vi "canDataSort.vi"() -> ()   [LabVIEW 2023] (continued)
\tFF\r\n      1212  1FFFFFFF   00000004    8        00\t20\tFF\tFF\tFF\tFF\tFF\tFF\r\n      1203  0CF102A7   00000004    8        30\t75\tE0\t2E\t80\tFF\tFF\tFD\r\n      1203  0CF101A7   00000004    8        68\t00\t97\tCC\t00\t15\t39\t56\r\n      1202  1FFFFFFF   00000004    8        00\t00\tFF\tFF\tFF\tFF\tFF\tFF\r\n      1243  0C3C4D4A   00000004    8        BE\tFF\tFF\t7F\t18\tFF\tFF\t44\r\n      1243  0CF101A7   00000004    8        68\t00\t97\tCC\t00\t16\t39\t58\r\n      1242  18F120F0   00000004    8        2B\t75\t60\tB1\tB0\t01\tFF\tFF\r\n      1241  18F11FF0   00000004    8        FF\t3F\t90\t68\t88\t1B\t10\t4C\r\n      1232  1FFFFFFF   00000004    8        00\t20\tFF\tFF\tFF\tFF\tFF\tFF\r\n      1223  0CF102A7   00000004    8        30\t75\tE0\t2E\t80\tFF\tFF\tFD\r\n      1223  0CF101A7   00000004    8        68\t00\t97\tCC\t00\t16\t39\t57\r\n      1222  1FFFFFFF   00000004    8        00\t00\tFF\tFF\tFF\tFF\tFF\tFF\r\n      1212  1FFFFFFF   00000004    8        00\t20\tFF\tFF\tFF\tFF\tFF\tFF\r\n      1203  0CF102A7   00000004    8        30\t75\tE0\t2E\t80\tFF\tFF\tFD\r\n      1203  0CF101A7   00000004    8        68\t00\t97\tCC\t00\t15\t39\t56\r\n      1244  0CF102A7   00000004    8        30\t75\tE0\t2E\t80\tFF\tFF\tFD\r\n      1243  0C3C4D4A   00000004    8        BE\tFF\tFF\t7F\t18\tFF\tFF\t44\r\n      1243  0CF101A7   00000004    8        68\t00\t97\tCC\t00\t16\t39\t58\r\n      1242  18F120F0   00000004    8        2B\t75\t60\tB1\tB0\t01\tFF\tFF\r\n      1241  18F11FF0   00000004    8        FF\t3F\t90\t68\t88\t1B\t10\t4C\r\n      1232  1FFFFFFF   00000004    8        00\t20\tFF\tFF\tFF\tFF\tFF\tFF\r\n      1223  0CF102A7   00000004    8        30\t75\tE0\t2E\t80\tFF\tFF\tFD\r\n      1223  0CF101A7   00000004    8        68\t00\t97\tCC\t00\t16\t39\t57\r\n      1222  1FFFFFFF   00000004    8        00\t00\tFF\tFF\tFF\tFF\tFF\tFF\r\n      1212  1FFFFFFF   00000004    8        00\t20\tFF\tFF\tFF\tFF\tFF\tFF\r\n      1203  0CF102A7   00000004    8        30\t75\tE0\t2E\t80\tFF\tFF\tFD\r\n      1244  0CF103A7   00000004    8        17\t1F\t08\t60\tB1\t1F\t08\t44\r\n      1244  0CF102A7   00000004    8        30\t75\tE0\t2E\t80\tFF\tFF\tFD\r\n      1243  0C3C4D4A   00000004    8        BE\tFF\tFF\t7F\t18\tFF\tFF\t44\r\n      1243  0CF101A7   00000004    8        68\t00\t97\tCC\t00\t16\t39\t58\r\n      1242  18F120F0   00000004    8        2B\t75\t60\tB1\tB0\t01\tFF\tFF\r\n      1241  18F11FF0   00000004    8        FF\t3F\t90\t68\t88\t1B\t10\t4C\r\n      1232  1FFFFFFF   00000004    8        00\t20\tFF\tFF\tFF\tFF\tFF\tFF\r\n      1223  0CF102A7   00000004    8        30\t75\tE0\t2E\t80\tFF\tFF\tFD\r\n      1223  0CF101A7   00000004    8        68\t00\t97\tCC\t00\t16\t39\t57\r\n      1222  1FFFFFFF   00000004    8        00\t00\tFF\tFF\tFF\tFF\tFF\tFF\r\n      1212  1FFFFFFF   00000004    8        00\t20\tFF\tFF\tFF\tFF\tFF\tFF\r\n      1245  0CF104A7   00000004    8        F0\t60\t22\tFC\tFF\tFF\tFF\t44\r\n      1244  0CF103A7   00000004    8        17\t1F\t08\t60\tB1\t1F\t08\t44\r\n      1244  0CF102A7   00000004    8        30\t75\tE0\t2E\t80\tFF\tFF\tFD\r\n      1243  0C3C4D4A   00000004    8        BE\tFF\tFF\t7F\t18\tFF\tFF\t44\r\n      1243  0CF101A7   00000004    8        68\t00\t97\tCC\t00\t16\t39\t58\r\n      1242  18F120F0   00000004    8        2B\t75\t60\tB1\tB0\t01\tFF\tFF\r\n      1241  18F11FF0   00000004    8        FF\t3F\t90\t68\t88\t1B\t10\t4C\r\n      1232  1FFFFFFF   00000004    8        00\t20\tFF\tFF\tFF\tFF\tFF\tFF\r\n      1223  0CF102A7   00000004    8        30\t75\tE0\t2E\t80\tFF\tFF\tFD\r\n      1223  0CF101A7   00000004    8        68\t00\t97\tCC\t00\t16\t39\t57\r\n      1222  1FFFFFFF   00000004    8        00\t00\tFF\tFF\tFF\tFF\tFF\tFF\r\n      1245  18F106A7   00000004    8        00\tF7\tFF\tFF\tFF\tFF\tFF\t89\r\n      1245  0CF104A7   00000004    8        F0\t60\t22\tFC\tFF\tFF\tFF\t44\r\n      1244  0CF103A7   00000004    8        17\t1F\t08\t60\tB1\t1F\t08\t44\r\n      1244  0CF102A7   00000004    8        30\t75\tE0\t2E\t80\tFF\tFF\tFD\r\n      1243  0C3C4D4A   00000004    8        BE\tFF\tFF\t7F\t18\tFF\tFF\t44\r\n      1243  0CF101A7   00000004    8        68\t00\t97\tCC\t00\t16\t39\t58\r\n      1242  18F120F0   00000004    8        2B\t75\t60\tB1\tB0\t01\tFF\tFF\r\n      1241  18F11FF0   00000004    8        FF\t3F\t90\t68\t88\t1B\t10\t4C\r\n      1232  1FFFFFFF   00000004    8        00\t20\tFF\tFF\tFF\tFF\tFF\tFF\r\n      1223  0CF102A7   00000004    8        30\t75\tE0\t2E\t80\tFF\tFF\tFD\r\n      1223  0CF101A7   00000004    8        68\t00\t97\tCC\t00\t16\t39\t57\r\n      1246  18F121F0   00000004    8        09\t18\t00\t00\tFF\tFF\tB0\t01\r\n      1245  18F106A7   00000004    8        00\tF7\tFF\tFF\tFF\tFF\tFF\t89\r\n      1245  0CF104A7   00000004    8        F0\t60\t22\tFC\tFF\tFF\tFF\t44\r\n      1244  0CF103A7   00000004    8        17\t1F\t08\t60\tB1\t1F\t08\t44\r\n      1244  0CF102A7   00000004    8        30\t75\tE0\t2E\t80\tFF\tFF\tFD\r\n      1243  0C3C4D4A   00000004    8        BE\tFF\tFF\t7F\t18\tFF\tFF\t44\r\n      1243  0CF101A7   00000004    8        68\t00\t97\tCC\t00\t16\t39\t58\r\n      1242  18F120F0   00000004    8        2B\t75\t60\tB1\tB0\t01\tFF\tFF\r\n      1241  18F11FF0   00000004    8        FF\t3F\t90\t68\t88\t1B\t10\t4C\r\n      1232  1FFFFFFF   00000004    8        00\t20\tFF\tFF\tFF\tFF\tFF\tFF\r\n      1223  0CF102A7   00000004    8        30\t75\tE0\t2E\t80\tFF\tFF\tFD\r\n      1247  1FFFFFFF   00000004    8        00\t20\tFF\tFF\tFF\tFF\tFF\tFF\r\n      1246  18F121F0   00000004    8        09\t18\t00\t00\tFF\tFF\tB0\t01\r\n      1245  18F106A7   00000004    8        00\tF7\tFF\tFF\tFF\tFF\tFF\t89\r\n      1245  0CF104A7   00000004    8        F0\t60\t22\tFC\tFF\tFF\tFF\t44\r\n      1244  0CF103A7   00000004    8        17\t1F\t08\t60\tB1\t1F\t08\t44\r\n      1244  0CF102A7   00000004    8        30\t75\tE0\t2E\t80\tFF\tFF\tFD\r\n      1243  0C3C4D4A   00000004    8        BE\tFF\tFF\t7F\t18\tFF\tFF\t44\r\n      1243  0CF101A7   00000004    8        68\t00\t97\tCC\t00\t16\t39\t58\r\n      1242  18F120F0   00000004    8        2B\t75\t60\tB1\tB0\t01\tFF\tFF\r\n      1241  18F11FF0   00000004    8        FF\t3F\t90\t68\t88\t1B\t10\t4C\r\n      1232  1FFFFFFF   00000004    8        00\t20\tFF\tFF\tFF\tFF\tFF\tFF\r\n      1252  1FFFFFFF   00000004    8        00\t20\tFF\tFF\tFF\tFF\tFF\tFF\r\n      1247  1FFFFFFF   00000004    8        00\t20\tFF\tFF\tFF\tFF\tFF\tFF\r\n      1246  18F121F0   00000004    8        09\t18\t00\t00\tFF\tFF\tB0\t01\r\n      1245  18F106A7   00000004    8        00\tF7\tFF\tFF\tFF\tFF\tFF\t89\r\n      1245  0CF104A7   00000004    8        F0\t60\t22\tFC\tFF\tFF\tFF\t44\r\n      1244  0CF103A7   00000004    8        17\t1F\t08\t60\tB1\t1F\t08\t44\r\n      1244  0CF102A7   00000004    8        30\t75\tE0\t2E\t80\tFF\tFF\tFD\r\n      1243  0C3C4D4A   00000004    8        BE\tFF\tFF\t7F\t18\tFF\tFF\t44\r\n      1243  0CF101A7   00000004    8        68\t00\t97\tCC\t00\t16\t39\t58\r\n      1242  18F120F0   00000004    8        2B\t75\t60\tB1\tB0\t01\tFF\tFF\r\n      1241  18F11FF0   00000004    8        FF\t3F\t90\t68\t88\t1B\t10\t4C\r\n      1262  1FFFFFFF   00000004    8        00\t00\tFF\tFF\tFF\tFF\tFF\tFF\r\n      1252  1FFFFFFF   00000004    8        00\t20\tFF\tFF\tFF\tFF\tFF\tFF\r\n      1247  1FFFFFFF   00000004    8        00\t20\tFF\tFF\tFF\tFF\tFF\tFF\r\n      1246  18F121F0   00000004    8        09\t18\t00\t00\tFF\tFF\tB0\t01\r\n      1245  18F106A7   00000004    8        00\tF7\tFF\tFF\tFF\tFF\tFF\t89\r\n      1245  0CF104A7   00000004    8        F0\t60\t22\tFC\tFF\tFF\tFF\t44\r\n      1244  0CF103A7   00000004    8        17\t1F\t08\t60\tB1\t1F\t08\t44\r\n      1244  0CF102A7   00000004    8        30\t75\tE0\t2E\t80\tFF\tFF\tFD\r\n      1243  0C3C4D4A   00000004    8        BE\tFF\tFF\t7F\t18\tFF\tFF\t44\r\n      1243  0CF101A7   00000004    8        68\t00\t97\tCC\t00\t16\t39\t58\r\n      1242  18F120F0   00000004    8        2B\t75\t60\tB1\tB0\t01\tFF\tFF\r\n      1263  0CF101A7   00000004    8        68\t00\t97\tCC\t00\t16\t39\t59\r\n      1262  1FFFFFFF   00000004    8        00\t00\tFF\tFF\tFF\tFF\tFF\tFF\r\n      1252  1FFFFFFF   00000004    8        00\t20\tFF\tFF\tFF\tFF\tFF\tFF\r\n      1247  1FFFFFFF   00000004    8        00\t20\tFF\tFF\tFF\tFF\tFF\tFF\r\n      1246  18F121F0   00000004    8        09\t18\t00\t00\tFF\tFF\tB0\t01\r\n      1245  18F106A7   00000004    8        00\tF7\tFF\tFF\tFF\tFF\tFF\t89\r\n      1245  0CF104A7   00000004    8        F0\t60\t22\tFC\tFF\tFF\tFF\t44\r\n      1244  0CF103A7   00000004    8        17\t1F\t08\t60\tB1\t1F\t08\t44\r\n      1244  0CF102A7   00000004    8        30\t75\tE0\t2E\t80\tFF\tFF\tFD\r\n      1243  0C3C4D4A   00000004    8        BE\tFF\tFF\t7F\t18\tFF\tFF\t44\r\n      1243  0CF101A7   00000004    8        68\t00\t97\tCC\t00\t16\t39\t58\r\n      1263  0CF102A7   00000004    8        30\t75\tE0\t2E\t80\tFF\tFF\tFD\r\n      1263  0CF101A7   00000004    8        68\t00\t97\tCC\t00\t16\t39\t59\r\n      1262  1FFFFFFF   00000004    8        00\t00\tFF\tFF\tFF\tFF\tFF\tFF\r\n      1252  1FFFFFFF   00000004    8        00\t20\tFF\tFF\tFF\tFF\tFF\tFF\r\n      1247  1FFFFFFF   00000004    8        00\t20\tFF\tFF\tFF\tFF\tFF\tFF\r\n      1246  18F121F0   00000004    8        09\t18\t00\t00\tFF\tFF\tB0\t01\r\n      1245  18F106A7   00000004    8        00\tF7\tFF\tFF\tFF\tFF\tFF\t89\r\n      1245  0CF104A7   00000004    8        F0\t60\t22\tFC\tFF\tFF\tFF\t44\r\n      1244  0CF103A7   00000004    8        17\t1F\t08\t60\tB1\t1F\t08\t44\r\n      1244  0CF102A7   00000004    8        30\t75\tE0\t2E\t80\tFF\tFF\tFD\r\n      1243  0C3C4D4A   00000004    8        BE\tFF\tFF\t7F\t18\tFF\tFF\t44\r\n      1272  1FFFFFFF   00000004    8        00\t20\tFF\tFF\tFF\tFF\tFF\tFF\r\n      1263  0CF102A7   00000004    8        30\t75\tE0\t2E\t80\tFF\tFF\tFD\r\n      1263  0CF101A7   00000004    8        68\t00\t97\tCC\t00\t16\t39\t59\r\n      1262  1FFFFFFF   00000004    8        00\t00\tFF\tFF\tFF\tFF\tFF\tFF\r\n      1252  1FFFFFFF   00000004    8        00\t20\tFF\tFF\tFF\tFF\tFF\tFF\r\n      1247  1FFFFFFF   00000004    8        00\t20\tFF\tFF\tFF\tFF\tFF\tFF\r\n      1246  18F121F0   00000004    8        09\t18\t00\t00\tFF\tFF\tB0\t01\r\n      1245  18F106A7   00000004    8        00\tF7\tFF\tFF\tFF\tFF\tFF\t89\r\n      1245  0CF104A7   00000004    8        F0\t60\t22\tFC\tFF\tFF\tFF\t44\r\n      1244  0CF103A7   00000004    8        17\t1F\t08\t60\tB1\t1F\t08\t44\r\n      1244  0CF102A7   00000004    8        30\t75\tE0\t2E\t80\tFF\tFF\tFD\r\n      1282  1FFFFFFF   00000004    8        00\t00\tFF\tFF\tFF\tFF\tFF\tFF\r\n      1272  1FFFFFFF   00000004    8        00\t20\tFF\tFF\tFF\tFF\tFF\tFF\r\n      1263  0CF102A7   00000004    8        30\t75\tE0\t2E\t80\tFF\tFF\tFD\r\n      1263  0CF101A7   00000004    8        68\t00\t97\tCC\t00\t16\t39\t59\r\n      1262  1FFFFFFF   00000004    8        00\t00\tFF\tFF\tFF\tFF\tFF\tFF\r\n      1252  1FFFFFFF   00000004    8        00\t20\tFF\tFF\tFF\tFF\tFF\tFF\r\n      1247  1FFFFFFF   00000004    8        00\t20\tFF\tFF\tFF\tFF\tFF\tFF\r\n      1246  18F121F0   00000004    8        09\t18\t00\t00\tFF\tFF\tB0\t01\r\n      1245  18F106A7   00000004    8        00\tF7\tFF\tFF\tFF\tFF\tFF\t89\r\n      1245  0CF104A7   00000004    8        F0\t60\t22\tFC\tFF\tFF\tFF\t44\r\n      1244  0CF103A7   00000004    8        17\t1F\t08\t60\tB1\t1F\t08\t44\r\n      1283  0CF101A7   00000004    8        68\t00\t97\tCC\t00\t16\t39\t5A\r\n      1282  1FFFFFFF   00000004    8        00\t00\tFF\tFF\tFF\tFF\tFF\tFF\r\n      1272  1FFFFFFF   00000004    8        00\t20\tFF\tFF\tFF\tFF\tFF\tFF\r\n      1263  0CF102A7   00000004    8        30\t75\tE0\t2E\t80\tFF\tFF\tFD\r\n      1263  0CF101A7   00000004    8        68\t00\t97\tCC\t00\t16\t39\t59\r\n      1262  1FFFFFFF   00000004    8        00\t00\tFF\tFF\tFF\tFF\tFF\tFF\r\n      1252  1FFFFFFF   00000004    8        00\t20\tFF\tFF\tFF\tFF\tFF\tFF\r\n      1247  1FFFFFFF   00000004    8        00\t20\tFF\tFF\tFF\tFF\tFF\tFF\r\n      1246  18F121F0   00000004    8        09\t18\t00\t00\tFF\tFF\tB0\t01\r\n      1245  18F106A7   00000004    8        00\tF7\tFF\tFF\tFF\tFF\tFF\t89\r\n      1245  0CF104A7   00000004    8        F0\t60\t22\tFC\tFF\tFF\tFF\t44\r\n      1283  0CF102A7   00000004    8        30\t75\tE0\t2E\t80\tFF\tFF\tFD\r\n      1283  0CF101A7   00000004    8        68\t00\t97\tCC\t00\t16\t39\t5A\r\n      1282  1FFFFFFF   00000004    8        00\t00\tFF\tFF\tFF\tFF\tFF\tFF\r\n      1272  1FFFFFFF   00000004    8        00\t20\tFF\tFF\tFF\tFF\tFF\tFF\r\n      1263  0CF102A7   00000004    8        30\t75\tE0\t2E\t80\tFF\tFF\tFD\r\n      1263  0CF101A7   00000004    8        68\t00\t97\tCC\t00\t16\t39\t59\r\n      1262  1FFFFFFF   00000004    8        00\t00\tFF\tFF\tFF\tFF\tFF\tFF\r\n      1252  1FFFFFFF   00000004    8        00\t20\tFF\tFF\tFF\tFF\tFF\tFF\r\n      1247  1FFFFFFF   00000004    8        00\t20\tFF\tFF\tFF\tFF\tFF\tFF\r\n      1246  18F121F0   00000004    8        09\t18\t00\t00\tFF\tFF\tB0\t01\r\n      1245  18F106A7   00000004    8        00\tF7\tFF\tFF\tFF\tFF\tFF\t89\r\n      1292  1FFFFFFF   00000004    8        00\t20\tFF\tFF\tFF\tFF\tFF\tFF\r\n      1283  0CF102A7   00000004    8        30\t75\tE0\t2E\t80\tFF\tFF\tFD\r\n      1283  0CF101A7   00000004    8        68\t00\t97\tCC\t00\t16\t39\t5A\r\n      1282  1FFFFFFF   00000004    8        00\t00\tFF\tFF\tFF\tFF\tFF\tFF\r\n      1272  1FFFFFFF   00000004    8        00\t20\tFF\tFF\tFF\tFF\tFF\tFF\r\n      1263  0CF102A7   00000004    8        30\t75\tE0\t2E\t80\tFF\tFF\tFD\r\n      1263  0CF101A7   00000004    8        68\t00\t97\tCC\t00\t16\t39\t59\r\n      1262  1FFFFFFF   00000004    8        00\t00\tFF\tFF\tFF\tFF\tFF\tFF\r\n      1252  1FFFFFFF   00000004    8        00\t20\tFF\tFF\tFF\tFF\tFF\tFF\r\n      1247  1FFFFFFF   00000004    8        00\t20\tFF\tFF\tFF\tFF\tFF\tFF\r\n      1246  18F121F0   00000004    8        09\t18\t00\t00\tFF\tFF\tB0\t01\r\n      1293  18F106A7   00000004    8        00\tF7\tFF\tFF\tFF\tFF\tFF\t8A\r\n      1292  1FFFFFFF   00000004    8        00\t20\tFF\tFF\tFF\tFF\tFF\tFF\r\n      1283  0CF102A7   00000004    8        30\t75\tE0\t2E\t80\tFF\tFF\tFD\r\n      1283  0CF101A7   00000004    8        68\t00\t97\tCC\t00\t16\t39\t5A\r\n      1282  1FFFFFFF   00000004    8        00\t00\tFF\tFF\tFF\tFF\tFF\tFF\r\n      1272  1FFFFFFF   00000004    8        00\t20\tFF\tFF\tFF\tFF\tFF\tFF\r\n      1263  0CF102A7   00000004    8        30\t75\tE0\t2E\t80\tFF\tFF\tFD\r\n      1263  0CF101A7   00000004    8        68\t00\t97\tCC\t00\t16\t39\t59\r\n      1262  1FFFFFFF   00000004    8        00\t00\tFF\tFF\tFF\tFF\tFF\tFF\r\n      1252  1FFFFFFF   00000004    8        00\t20\tFF\tFF\tFF\tFF\tFF\tFF\r\n      1247  1FFFFFFF   00000004    8        00\t20\tFF\tFF\tFF\tFF\tFF\tFF\r\n      1302  1FFFFFFF   00000004    8        00\t00\tFF\tFF\tFF\tFF\tFF\tFF\r\n      1293  18F106A7   00000004    8        00\tF7\tFF\tFF\tFF\tFF\tFF\t8A\r\n      1292  1FFFFFFF   00000004    8        00\t20\tFF\tFF\tFF\tFF\tFF\tFF\r\n      1283  0CF102A7   00000004    8        30\t75\tE0\t2E\t80\tFF\tFF\tFD\r\n      1283  0CF101A7   00000004    8        68\t00\t97\tCC\t00\t16\t39\t5A\r\n      1282  1FFFFFFF   00000004    8        00\t00\tFF\tFF\tFF\tFF\tFF\tFF\r\n      1272  1FFFFFFF   00000004    8        00\t20\tFF\tFF\tFF\tFF\tFF\tFF\r\n      1263  0CF102A7   00000004    8        30\t75\tE0\t2E\t80\tFF\tFF\tFD\r\n      1263  0CF101A7   00000004    8        68\t00\t97\tCC\t00\t16\t39\t59\r\n      1262  1FFFFFFF   00000004    8        00\t00\tFF\tFF\tFF\tFF\tFF\tFF\r\n      1252  1FFFFFFF   00000004    8        00\t20\tFF\tFF\tFF\tFF\tFF\tFF\r\n      1303  0CF101A7   00000004    8        68\t00\t97\tCC\t00\t16\t39\t5B\r\n      1302  1FFFFFFF   00000004    8        00\t00\tFF\tFF\tFF\tFF\tFF\tFF\r\n      1293  18F106A7   00000004    8        00\tF7\tFF\tFF\tFF\tFF\tFF\t8A\r\n      1292  1FFFFFFF   00000004    8        00\t20\tFF\tFF\tFF\tFF\tFF\tFF\r\n      1283  0CF102A7   00000004    8        30\t75\tE0\t2E\t80\tFF\tFF\tFD\r\n      1283  0CF101A7   00000004    8        68\t00\t97\tCC\t00\t16\t39\t5A\r\n      1282  1FFFFFFF   00000004    8        00\t00\tFF\tFF\tFF\tFF\tFF\tFF\r\n      1272  1FFFFFFF   00000004    8        00\t20\tFF\tFF\tFF\tFF\tFF\tFF\r\n      1263  0CF102A7   00000004    8        30\t75\tE0\t2E\t80\tFF\tFF\tFD\r\n      1263  0CF101A7   00000004    8        68\t00\t97\tCC\t00\t16\t39\t59\r\n      1262  1FFFFFFF   00000004    8        00\t00\tFF\tFF\tFF\tFF\tFF\tFF\r\n      1303  0CF102A7   00000004    8        30\t75\tE0\t2E\t80\tFF\tFF\tFD\r\n      1303  0CF101A7   00000004    8        68\t00\t97\tCC\t00\t16\t39\t5B\r\n      1302  1FFFFFFF   00000004    8        00\t00\tFF\tFF\tFF\tFF\tFF\tFF\r\n      1293  18F106A7   00000004    8        00\tF7\tFF\tFF\tFF\tFF\tFF\t8A\r\n      1292  1FFFFFFF   00000004    8        00\t20\tFF\tFF\tFF\tFF\tFF\tFF\r\n      1283  0CF102A7   00000004    8        30\t75\tE0\t2E\t80\tFF\tFF\tFD\r\n      1283  0CF101A7   00000004    8        68\t00\t97\tCC\t00\t16\t39\t5A\r\n      1282  1FFFFFFF   00000004    8        00\t00\tFF\tFF\tFF\tFF\tFF\tFF\r\n      1272  1FFFFFFF   00000004    8        00\t20\tFF\tFF\tFF\tFF\tFF\tFF\r\n      1263  0CF102A7   00000004    8        30\t75\tE0\t2E\t80\tFF\tFF\tFD\r\n      1263  0CF101A7   00000004    8        68\t00\t97\tCC\t00\t16\t39\t59\r\n      1312  1FFFFFFF   00000004    8        00\t20\tFF\tFF\tFF\tFF\tFF\tFF\r\n      1303  0CF102A7   00000004    8        30\t75\tE0\t2E\t80\tFF\tFF\tFD\r\n      1303  0CF101A7   00000004    8        68\t00\t97\tCC\t00\t16\t39\t5B\r\n      1302  1FFFFFFF   00000004    8        00\t00\tFF\tFF\tFF\tFF\tFF\tFF\r\n      1293  18F106A7   00000004    8        00\tF7\tFF\tFF\tFF\tFF\tFF\t8A\r\n      1292  1FFFFFFF   00000004    8        00\t20\tFF\tFF\tFF\tFF\tFF\tFF\r\n      1283  0CF102A7   00000004    8        30\t75\tE0\t2E\t80\tFF\tFF\tFD\r\n      1283  0CF101A7   00000004    8        68\t00\t97\tCC\t00\t16\t39\t5A\r\n      1282  1FFFFFFF   00000004    8        00\t00\tFF\tFF\tFF\tFF\tFF\tFF\r\n      1272  1FFFFFFF   00000004    8        00\t20\tFF\tFF\tFF\tFF\tFF\tFF\r\n      1263  0CF102A7   00000004    8        30\t75\tE0\t2E\t80\tFF\tFF\tFD\r\n      1322  1FFFFFFF   00000004    8        00\t00\tFF\tFF\tFF\tFF\tFF\tFF\r\n      1312  1FFFFFFF   00000004    8        00\t20\tFF\tFF\tFF\tFF\tFF\tFF\r\n      1303  0CF102A7   00000004    8        30\t75\tE0\t2E\t80\tFF\tFF\tFD\r\n      1303  0CF101A7   00000004    8        68\t00\t97\tCC\t00\t16\t39\t5B\r\n      1302  1FFFFFFF   00000004    8        00\t00\tFF\tFF\tFF\tFF\tFF\tFF\r\n      1293  18F106A7   00000004    8        00\tF7\tFF\tFF\tFF\tFF\tFF\t8A\r\n      1292  1FFFFFFF   00000004    8        00\t20\tFF\tFF\tFF\tFF\tFF\tFF\r\n      1283  0CF102A7   00000004    8        30\t75\tE0\t2E\t80\tFF\tFF\tFD\r\n      1283  0CF101A7   00000004    8        68\t00\t97\tCC\t00\t16\t39\t5A\r\n      1282  1FFFFFFF   00000004    8        00\t00\tFF\tFF\tFF\tFF\tFF\tFF\r\n      1272  1FFFFFFF   00000004    8        00\t20\tFF\tFF\tFF\tFF\tFF\tFF\r\n      1323  0CF101A7   00000004    8        68\t00\t97\tCC\t00\t16\t39\t5C\r\n      1322  1FFFFFFF   00000004    8        00\t00\tFF\tFF\tFF\tFF\tFF\tFF\r\n      1312  1FFFFFFF   00000004    8        00\t20\tFF\tFF\tFF\tFF\tFF\tFF\r\n      1303  0CF102A7   00000004    8        30\t75\tE0\t2E\t80\tFF\tFF\tFD\r\n      1303  0CF101A7   00000004    8        68\t00\t97\tCC\t00\t16\t39\t5B\r\n      1302  1FFFFFFF   00000004    8        00\t00\tFF\tFF\tFF\tFF\tFF\tFF\r\n      1293  18F106A7   00000004    8        00\tF7\tFF\tFF\tFF\tFF\tFF\t8A\r\n      1292  1FFFFFFF   00000004    8        00\t20\tFF\tFF\tFF\tFF\tFF\tFF\r\n      1283  0CF102A7   00000004    8        30\t75\tE0\t2E\t80\tFF\tFF\tFD\r\n      1283  0CF101A7   00000004    8        68\t00\t97\tCC\t00\t16\t39\t5A\r\n      1282  1FFFFFFF   00000004    8        00\t00\tFF\tFF\tFF\tFF\tFF\tFF\r\n      1323  0CF102A7   00000004    8        30\t75\tE0\t2E\t80\tFF\tFF\tFD\r\n      1323  0CF101A7   00000004    8        68\t00\t97\tCC\t00\t16\t39\t5C\r\n      1322  1FFFFFFF   00000004    8        00\t00\tFF\tFF\tFF\tFF\tFF\tFF\r\n      1312  1FFFFFFF   00000004    8        00\t20\tFF\tFF\tFF\tFF\tFF\tFF\r\n      1303  0CF102A7   00000004    8        30\t75\tE0\t2E\t80\tFF\tFF\tFD\r\n      1303  0CF101A7   00000004    8        68\t00\t97\tCC\t00\t16\t39\t5B\r\n      1302  1FFFFFFF   00000004    8        00\t00\tFF\tFF\tFF\tFF\tFF\tFF\r\n      1293  18F106A7   00000004    8        00\tF7\tFF\tFF\tFF\tFF\tFF\t8A\r\n      1292  1FFFFFFF   00000004    8        00\t20\tFF\tFF\tFF\tFF\tFF\tFF\r\n      1283  0CF102A7   00000004    8        30\t75\tE0\t2E\t80\tFF\tFF\tFD\r\n      1283  0CF101A7   00000004    8        68\t00\t97\tCC\t00\t16\t39\t5A\r\n      1332  1FFFFFFF   00000004    8        00\t20\tFF\tFF\tFF\tFF\tFF\tFF\r\n      1323  0CF102A7   00000004    8        30\t75\tE0\t2E\t80\tFF\tFF\tFD\r\n      1323  0CF101A7   00000004    8        68\t00\t97\tCC\t00\t16\t39\t5C\r\n      1322  1FFFFFFF   00000004    8        00\t00\tFF\tFF\tFF\tFF\tFF\tFF\r\n      1312  1FFFFFFF   00000004    8        00\t20\tFF\tFF\tFF\tFF\tFF\tFF\r\n      1303  0CF102A7   00000004    8        30\t75\tE0\t2E\t80\tFF\tFF\tFD\r\n      1303  0CF101A7   00000004    8        68\t00\t97\tCC\t00\t16\t39\t5B\r\n      1302  1FFFFFFF   00000004    8        00\t00\tFF\tFF\tFF\tFF\tFF\tFF\r\n      1293  18F106A7   00000004    8        00\tF7\tFF\tFF\tFF\tFF\tFF\t8A\r\n      1292  1FFFFFFF   00000004    8        00\t20\tFF\tFF\tFF\tFF\tFF\tFF\r\n      1283  0CF102A7   00000004    8        30\t75\tE0\t2E\t80\tFF\tFF\tFD\r\n      1341  18F11FF0   00000004    8        FF\t3F\t90\t68\t88\t1B\t10\t5C\r\n      1332  1FFFFFFF   00000004    8        00\t20\tFF\tFF\tFF\tFF\tFF\tFF\r\n      1323  0CF102A7   00000004    8        30\t75\tE0\t2E\t80\tFF\tFF\tFD\r\n      1323  0CF101A7   00000004    8        68\t00\t97\tCC\t00\t16\t39\t5C\r\n      1322  1FFFFFFF   00000004    8        00\t00\tFF\tFF\tFF\tFF\tFF\tFF\r\n      1312  1FFFFFFF   00000004    8        00\t20\tFF\tFF\tFF\tFF\tFF\tFF\r\n      1303  0CF102A7   00000004    8        30\t75\tE0\t2E\t80\tFF\tFF\tFD\r\n      1303  0CF101A7   00000004    8        68\t00\t97\tCC\t00\t16\t39\t5B\r\n      1302  1FFFFFFF   00000004    8        00\t00\tFF\tFF\tFF\tFF\tFF\tFF\r\n      1293  18F106A7   00000004    8        00\tF7\tFF\tFF\tFF\tFF\tFF\t8A\r\n      1292  1FFFFFFF   00000004    8        00\t20\tFF\tFF\tFF\tFF\tFF\tFF\r\n      1342  18F120F0   00000004    8        2B\t75\t60\tB1\tB0\t01\tFF\tFF\r\n      1341  18F11FF0   00000004    8        FF\t3F\t90\t68\t88\t1B\t10\t5C\r\n      1332  1FFFFFFF   00000004    8        00\t20\tFF\tFF\tFF\tFF\tFF\tFF\r\n      1323  0CF102A7   00000004    8        30\t75\tE0\t2E\t80\tFF\tFF\tFD\r\n      1323  0CF101A7   00000004    8        68\t00\t97\tCC\t00\t16\t39\t5C\r\n      1322  1FFFFFFF   00000004    8        00\t00\tFF\tFF\tFF\tFF\tFF\tFF\r\n      1312  1FFFFFFF   00000004    8        00\t20\tFF\tFF\tFF\tFF\tFF\tFF\r\n      1303  0CF102A7   00000004    8        30\t75\tE0\t2E\t80\tFF\tFF\tFD\r\n      1303  0CF101A7   00000004    8        68\t00\t97\tCC\t00\t16\t39\t5B\r\n      1302  1FFFFFFF   00000004    8        00\t00\tFF\tFF\tFF\tFF\tFF\tFF\r\n      1293  18F106A7   00000004    8        00\tF7\tFF\tFF\tFF\tFF\tFF\t8A\r\n      1343  0CF101A7   00000004    8        68\t00\t97\tCC\t00\t16\t39\t5D\r\n      1342  18F120F0   00000004    8        2B\t75\t60\tB1\tB0\t01\tFF\tFF\r\n      1341  18F11FF0   00000004    8        FF\t3F\t90\t68\t88\t1B\t10\t5C\r\n      1332  1FFFFFFF   00000004    8        00\t20\tFF\tFF\tFF\tFF\tFF\tFF\r\n      1323  0CF102A7   00000004    8        30\t75\tE0\t2E\t80\tFF\tFF\tFD\r\n      1323  0CF101A7   00000004    8        68\t00\t97\tCC\t00\t16\t39\t5C\r\n      1322  1FFFFFFF   00000004    8        00\t00\tFF\tFF\tFF\tFF\tFF\tFF\r\n      1312  1FFFFFFF   00000004    8        00\t20\tFF\tFF\tFF\tFF\tFF\tFF\r\n      1303  0CF102A7   00000004    8        30\t75\tE0\t2E\t80\tFF\tFF\tFD\r\n      1303  0CF101A7   00000004    8        68\t00\t97\tCC\t00\t16\t39\t5B\r\n      1302  1FFFFFFF   00000004    8        00\t00\tFF\tFF\tFF\tFF\tFF\tFF\r\n      1343  0C3C4D4A   00000004    8        BE\tFF\tFF\t7F\t18\tFF\tFF\t45\r\n      1343  0CF101A7   00000004    8        68\t00\t97\tCC\t00\t16\t39\t5D\r\n      1342  18F120F0   00000004    8        2B\t75\t60\tB1\tB0\t01\tFF\tFF\r\n      1341  18F11FF0   00000004    8        FF\t3F\t90\t68\t88\t1B\t10\t5C\r\n      1332  1FFFFFFF   00000004    8        00\t20\tFF\tFF\tFF\tFF\tFF\tFF\r\n      1323  0CF102A7   00000004    8        30\t75\tE0\t2E\t80\tFF\tFF\tFD\r\n      1323  0CF101A7   00000004    8        68\t00\t97\tCC\t00\t16\t39\t5C\r\n      1322  1FFFFFFF   00000004    8        00\t00\tFF\tFF\tFF\tFF\tFF\tFF\r\n      1312  1FFFFFFF   00000004    8        00\t20\tFF\tFF\tFF\tFF\tFF\tFF\r\n      1303  0CF102A7   00000004    8        30\t75\tE0\t2E\t80\tFF\tFF\tFD\r\n      1303  0CF101A7   00000004    8        68\t00\t97\tCC\t00\t16\t39\t5B\r\n      1344  0CF102A7   00000004    8        30\t75\tE0\t2E\t80\tFF\tFF\tFD\r\n      1343  0C3C4D4A   00000004    8        BE\tFF\tFF\t7F\t18\tFF\tFF\t45\r\n      1343  0CF101A7   00000004    8        68\t00\t97\tCC\t00\t16\t39\t5D\r\n      1342  18F120F0   00000004    8        2B\t75\t60\tB1\tB0\t01\tFF\tFF\r\n      1341  18F11FF0   00000004    8        FF\t3F\t90\t68\t88\t1B\t10\t5C\r\n      1332  1FFFFFFF   00000004    8        00\t20\tFF\tFF\tFF\tFF\tFF\tFF\r\n      1323  0CF102A7   00000004    8        30\t75\tE0\t2E\t80\tFF\tFF\tFD\r\n      1323  0CF101A7   00000004    8        68\t00\t97\tCC\t00\t16\t39\t5C\r\n      1322  1FFFFFFF   00000004    8        00\t00\tFF\tFF\tFF\tFF\tFF\tFF\r\n      1312  1FFFFFFF   00000004    8        00\t20\tFF\tFF\tFF\tFF\tFF\tFF\r\n      1303  0CF102A7   00000004    8        30\t75\tE0\t2E\t80\tFF\tFF\tFD\r\n      1344  0CF103A7   00000004    8        17\t1F\t08\t60\tB1\t1F\t08\t45\r\n      1344  0CF102A7   00000004    8        30\t75\tE0\t2E\t80\tFF\tFF\tFD\r\n      1343  0C3C4D4A   00000004    8        BE\tFF\tFF\t7F\t18\tFF\tFF\t45\r\n      1343  0CF101A7   00000004    8        68\t00\t97\tCC\t00\t16\t39\t5D\r\n      1342  18F120F0   00000004    8        2B\t75\t60\tB1\tB0\t01\tFF\tFF\r\n      1341  18F11FF0   00000004    8        FF\t3F\t90\t68\t88\t1B\t10\t5C\r\n      1332  1FFFFFFF   00000004    8        00\t20\tFF\tFF\tFF\tFF\tFF\tFF\r\n      1323  0CF102A7   00000004    8        30\t75\tE0\t2E\t80\tFF\tFF\tFD\r\n      1323  0CF101A7   00000004    8        68\t00\t97\tCC\t00\t16\t39\t5C\r\n      1322  1FFFFFFF   00000004    8        00\t00\tFF\tFF\tFF\tFF\tFF\tFF\r\n      1312  1FFFFFFF   00000004    8        00\t20\tFF\tFF\tFF\tFF\tFF\tFF\r\n      1345  0CF104A7   00000004    8        F0\t60\t22\tFC\tFF\tFF\tFF\t45\r\n      1344  0CF103A7   00000004    8        17\t1F\t08\t60\tB1\t1F\t08\t45\r\n      1344  0CF102A7   00000004    8        30\t75\tE0\t2E\t80\tFF\tFF\tFD\r\n      1343  0C3C4D4A   00000004    8        BE\tFF\tFF\t7F\t18\tFF\tFF\t45\r\n      1343  0CF101A7   00000004    8        68\t00\t97\tCC\t00\t16\t39\t5D\r\n      1342  18F120F0   00000004    8        2B\t75\t60\tB1\tB0\t01\tFF\tFF\r\n      1341  18F11FF0   00000004    8        FF\t3F\t90\t68\t88\t1B\t10\t5C\r\n      1332  1FFFFFFF   00000004    8        00\t20\tFF\tFF\tFF\tFF\tFF\tFF\r\n      1323  0CF102A7   00000004    8        30\t75\tE0\t2E\t80\tFF\tFF\tFD\r\n      1323  0CF101A7   00000004    8        68\t00\t97\tCC\t00\t16\t39\t5C\r\n      1322  1FFFFFFF   00000004    8        00\t00\tFF\tFF\tFF\tFF\tFF\tFF\r\n      1345  18F106A7   00000004    8        00\tF7\tFF\tFF\tFF\tFF\tFF\t8B\r\n      1345  0CF104A7   00000004    8        F0\t60\t22\tFC\tFF\tFF\tFF\t45\r\n      1344  0CF103A7   00000004    8        17\t1F\t08\t60\tB1\t1F\t08\t45\r\n      1344  0CF102A7   00000004    8        30\t75\tE0\t2E\t80\tFF\tFF\tFD\r\n      1343  0C3C4D4A   00000004    8        BE\tFF\tFF\t7F\t18\tFF\tFF\t45\r\n      1343  0CF101A7   00000004    8        68\t00\t97\tCC\t00\t16\t39\t5D\r\n      1342  18F120F0   00000004    8        2B\t75\t60\tB1\tB0\t01\tFF\tFF\r\n      1341  18F11FF0   00000004    8        FF\t3F\t90\t68\t88\t1B\t10\t5C\r\n      1332  1FFFFFFF   00000004    8        00\t20\tFF\tFF\tFF\tFF\tFF\tFF\r\n      1323  0CF102A7   00000004    8        30\t75\tE0\t2E\t80\tFF\tFF\tFD\r\n      1323  0CF101A7   00000004    8        68\t00\t97\tCC\t00\t16\t39\t5C\r\n      1346  18F121F0   00000004    8        09\t18\t00\t00\tFF\tFF\tB0\t01\r\n      1345  18F106A7   00000004    8        00\tF7\tFF\tFF\tFF\tFF\tFF\t8B\r\n      1345  0CF104A7   00000004    8        F0\t60\t22\tFC\tFF\tFF\tFF\t45\r\n      1344  0CF103A7   00000004    8        17\t1F\t08\t60\tB1\t1F\t08\t45\r\n      1344  0CF102A7   00000004    8        30\t75\tE0\t2E\t80\tFF\tFF\tFD\r\n      1343  0C3C4D4A   00000004    8        BE\tFF\tFF\t7F\t18\tFF\tFF\t45\r\n      1343  0CF101A7   00000004    8        68\t00\t97\tCC\t00\t16\t39\t5D\r\n      1342  18F120F0   00000004    8        2B\t75\t60\tB1\tB0\t01\tFF\tFF\r\n      1341  18F11FF0   00000004    8        FF\t3F\t90\t68\t88\t1B\t10\t5C\r\n      1332  1FFFFFFF   00000004    8        00\t20\tFF\tFF\tFF\tFF\tFF\tFF\r\n      1323  0CF102A7   00000004    8        30\t75\tE0\t2E\t80\tFF\tFF\tFD\r\n      1347  1FFFFFFF   00000004    8        00\t20\tFF\tFF\tFF\tFF\tFF\tFF\r\n      1346  18F121F0   00000004    8        09\t18\t00\t00\tFF\tFF\tB0\t01\r\n      1345  18F106A7   00000004    8        00\tF7\tFF\tFF\tFF\tFF\tFF\t8B\r\n      1345  0CF104A7   00000004    8        F0\t60\t22\tFC\tFF\tFF\tFF\t45\r\n      1344  0CF103A7   00000004    8        17\t1F\t08\t60\tB1\t1F\t08\t45\r\n      1344  0CF102A7   00000004    8        30\t75\tE0\t2E\t80\tFF\tFF\tFD\r\n      1343  0C3C4D4A   00000004    8        BE\tFF\tFF\t7F\t18\tFF\tFF\t45\r\n      1343  0CF101A7   00000004    8        68\t00\t97\tCC\t00\t16\t39\t5D\r\n      1342  18F120F0   00000004    8        2B\t75\t60\tB1\tB0\t01\tFF\tFF\r\n      1341  18F11FF0   00000004    8        FF\t3F\t90\t68\t88\t1B\t10\t5C\r\n      1332  1FFFFFFF   00000004    8        00\t20\tFF\tFF\tFF\tFF\tFF\tFF\r\n      1352  1FFFFFFF   00000004    8        00\t00\tFF\tFF\tFF\tFF\tFF\tFF\r\n      1347  1FFFFFFF   00000004    8        00\t20\tFF\tFF\tFF\tFF\tFF\tFF\r\n      1346  18F121F0   00000004    8        09\t18\t00\t00\tFF\tFF\tB0\t01\r\n      1345  18F106A7   00000004    8        00\tF7\tFF\tFF\tFF\tFF\tFF\t8B\r\n      1345  0CF104A7   00000004    8        F0\t60\t22\tFC\tFF\tFF\tFF\t45\r\n      1344  0CF103A7   00000004    8        17\t1F\t08\t60\tB1\t1F\t08\t45\r\n      1344  0CF102A7   00000004    8        30\t75\tE0\t2E\t80\tFF\tFF\tFD\r\n      1343  0C3C4D4A   00000004    8        BE\tFF\tFF\t7F\t18\tFF\tFF\t45\r\n      1343  0CF101A7   00000004    8        68\t00\t97\tCC\t00\t16\t39\t5D\r\n      1342  18F120F0   00000004    8        2B\t75\t60\tB1\tB0\t01\tFF\tFF\r\n      1341  18F11FF0   00000004    8        FF\t3F\t90\t68\t88\t1B\t10\t5C\r\n      1362  1FFFFFFF   00000004    8        00\t00\tFF\tFF\tFF\tFF\tFF\tFF\r\n      1352  1FFFFFFF   00000004    8        00\t00\tFF\tFF\tFF\tFF\tFF\tFF\r\n      1347  1FFFFFFF   00000004    8        00\t20\tFF\tFF\tFF\tFF\tFF\tFF\r\n      1346  18F121F0   00000004    8        09\t18\t00\t00\tFF\tFF\tB0\t01\r\n      1345  18F106A7   00000004    8        00\tF7\tFF\tFF\tFF\tFF\tFF\t8B\r\n      1345  0CF104A7   00000004    8        F0\t60\t22\tFC\tFF\tFF\tFF\t45\r\n      1344  0CF103A7   00000004    8        17\t1F\t08\t60\tB1\t1F\t08\t45\r\n      1344  0CF102A7   00000004    8        30\t75\tE0\t2E\t80\tFF\tFF\tFD\r\n      1343  0C3C4D4A   00000004    8        BE\tFF\tFF\t7F\t18\tFF\tFF\t45\r\n      1343  0CF101A7   00000004    8        68\t00\t97\tCC\t00\t16\t39\t5D\r\n      1342  18F120F0   00000004    8        2B\t75\t60\tB1\tB0\t01\tFF\tFF\r\n      1363  0CF101A7   00000004    8        68\t00\t97\tCC\t00\t16\t39\t5E\r\n      1362  1FFFFFFF   00000004    8        00\t00\tFF\tFF\tFF\tFF\tFF\tFF\r\n      1352  1FFFFFFF   00000004    8        00\t00\tFF\tFF\tFF\tFF\tFF\tFF\r\n      1347  1FFFFFFF   00000004    8        00\t20\tFF\tFF\tFF\tFF\tFF\tFF\r\n      1346  18F121F0   00000004    8        09\t18\t00\t00\tFF\tFF\tB0\t01\r\n      1345  18F106A7   00000004    8        00\tF7\tFF\tFF\tFF\tFF\tFF\t8B\r\n      1345  0CF104A7   00000004    8        F0\t60\t22\tFC\tFF\tFF\tFF\t45\r\n      1344  0CF103A7   00000004    8        17\t1F\t08\t60\tB1\t1F\t08\t45\r\n      1344  0CF102A7   00000004    8        30\t75\tE0\t2E\t80\tFF\tFF\tFD\r\n      1343  0C3C4D4A   00000004    8        BE\tFF\tFF\t7F\t18\tFF\tFF\t45\r\n      1343  0CF101A7   00000004    8        68\t00\t97\tCC\t00\t16\t39\t5D\r\n      1363  0CF102A7   00000004    8        30\t75\tE0\t2E\t80\tFF\tFF\tFD\r\n      1363  0CF101A7   00000004    8        68\t00\t97\tCC\t00\t16\t39\t5E\r\n      1362  1FFFFFFF   00000004    8        00\t00\tFF\tFF\tFF\tFF\tFF\tFF\r\n      1352  1FFFFFFF   00000004    8        00\t00\tFF\tFF\tFF\tFF\tFF\tFF\r\n      1347  1FFFFFFF   00000004    8        00\t20\tFF\tFF\tFF\tFF\tFF\tFF\r\n      1346  18F121F0   00000004    8        09\t18\t00\t00\tFF\tFF\tB0\t01\r\n      1345  18F106A7   00000004    8        00\tF7\tFF\tFF\tFF\tFF\tFF\t8B\r\n      1345  0CF104A7   00000004    8        F0\t60\t22\tFC\tFF\tFF\tFF\t45\r\n      1344  0CF103A7   00000004    8        17\t1F\t08\t60\tB1\t1F\t08\t45\r\n      1344  0CF102A7   00000004    8        30\t75\tE0\t2E\t80\tFF\tFF\tFD\r\n      1343  0C3C4D4A   00000004    8        BE\tFF\tFF\t7F\t18\tFF\tFF\t45\r\n      1372  1FFFFFFF   00000004    8        00\t00\tFF\tFF\tFF\tFF\tFF\tFF\r\n      1363  0CF102A7   00000004    8        30\t75\tE0\t2E\t80\tFF\tFF\tFD\r\n      1363  0CF101A7   00000004    8        68\t00\t97\tCC\t00\t16\t39\t5E\r\n      1362  1FFFFFFF   00000004    8        00\t00\tFF\tFF\tFF\tFF\tFF\tFF\r\n      1352  1FFFFFFF   00000004    8        00\t00\tFF\tFF\tFF\tFF\tFF\tFF\r\n      1347  1FFFFFFF   00000004    8        00\t20\tFF\tFF\tFF\tFF\tFF\tFF\r\n      1346  18F121F0   00000004    8        09\t18\t00\t00\tFF\tFF\tB0\t01\r\n      1345  18F106A7   00000004    8        00\tF7\tFF\tFF\tFF\tFF\tFF\t8B\r\n      1345  0CF104A7   00000004    8        F0\t60\t22\tFC\tFF\tFF\tFF\t45\r\n      1344  0CF103A7   00000004    8        17\t1F\t08\t60\tB1\t1F\t08\t45\r\n      1344  0CF102A7   00000004    8        30\t75\tE0\t2E\t80\tFF\tFF\tFD\r\n      1382  1FFFFFFF   00000004    8        00\t00\tFF\tFF\tFF\tFF\tFF\tFF\r\n      1372  1FFFFFFF   00000004    8        00\t00\tFF\tFF\tFF\tFF\tFF\tFF\r\n      1363  0CF102A7   00000004    8        30\t75\tE0\t2E\t80\tFF\tFF\tFD\r\n      1363  0CF101A7   00000004    8        68\t00\t97\tCC\t00\t16\t39\t5E\r\n      1362  1FFFFFFF   00000004    8        00\t00\tFF\tFF\tFF\tFF\tFF\tFF\r\n      1352  1FFFFFFF   00000004    8        00\t00\tFF\tFF\tFF\tFF\tFF\tFF\r\n      1347  1FFFFFFF   00000004    8        00\t20\tFF\tFF\tFF\tFF\tFF\tFF\r\n      1346  18F121F0   00000004    8        09\t18\t00\t00\tFF\tFF\tB0\t01\r\n      1345  18F106A7   00000004    8        00\tF7\tFF\tFF\tFF\tFF\tFF\t8B\r\n      1345  0CF104A7   00000004    8        F0\t60\t22\tFC\tFF\tFF\tFF\t45\r\n      1344  0CF103A7   00000004    8        17\t1F\t08\t60\tB1\t1F\t08\t45\r\n      1383  0CF101A7   00000004    8        68\t00\t97\tCC\t00\t16\t39\t5F\r\n      1382  1FFFFFFF   00000004    8        00\t00\tFF\tFF\tFF\tFF\tFF\tFF\r\n      1372  1FFFFFFF   00000004    8        00\t00\tFF\tFF\tFF\tFF\tFF\tFF\r\n      1363  0CF102A7   00000004    8        30\t75\tE0\t2E\t80\tFF\tFF\tFD\r\n      1363  0CF101A7   00000004    8        68\t00\t97\tCC\t00\t16\t39\t5E\r\n      1362  1FFFFFFF   00000004    8        00\t00\tFF\tFF\tFF\tFF\tFF\tFF\r\n      1352  1FFFFFFF   00000004    8        00\t00\tFF\tFF\tFF\tFF\tFF\tFF\r\n      1347  1FFFFFFF   00000004    8        00\t20\tFF\tFF\tFF\tFF\tFF\tFF\r\n      1346  18F121F0   00000004    8        09\t18\t00\t00\tFF\tFF\tB0\t01\r\n      1345  18F106A7   00000004    8        00\tF7\tFF\tFF\tFF\tFF\tFF\t8B\r\n      1345  0CF104A7   00000004    8        F0\t60\t22\tFC\tFF\tFF\tFF\t45\r\n      1383  0CF102A7   00000004    8        30\t75\tE0\t2E\t80\tFF\tFF\tFD\r\n      1383  0CF101A7   00000004    8        68\t00\t97\tCC\t00\t16\t39\t5F\r\n      1382  1FFFFFFF   00000004    8        00\t00\tFF\tFF\tFF\tFF\tFF\tFF\r\n      1372  1FFFFFFF   00000004    8        00\t00\tFF\tFF\tFF\tFF\tFF\tFF\r\n      1363  0CF102A7   00000004    8        30\t75\tE0\t2E\t80\tFF\tFF\tFD\r\n      1363  0CF101A7   00000004    8        68\t00\t97\tCC\t00\t16\t39\t5E\r\n      1362  1FFFFFFF   00000004    8        00\t00\tFF\tFF\tFF\tFF\tFF\tFF\r\n      1352  1FFFFFFF   00000004    8        00\t00\tFF\tFF\tFF\tFF\tFF\tFF\r\n      1347  1FFFFFFF   00000004    8        00\t20\tFF\tFF\tFF\tFF\tFF\tFF\r\n      1346  18F121F0   00000004    8        09\t18\t00\t00\tFF\tFF\tB0\t01\r\n      1345  18F106A7   00000004    8        00\tF7\tFF\tFF\tFF\tFF\tFF\t8B\r\n      1392  1FFFFFFF   00000004    8        00\t00\tFF\tFF\tFF\tFF\tFF\tFF\r\n      1383  0CF102A7   00000004    8        30\t75\tE0\t2E\t80\tFF\tFF\tFD\r\n      1383  0CF101A7   00000004    8        68\t00\t97\tCC\t00\t16\t39\t5F\r\n      1382  1FFFFFFF   00000004    8        00\t00\tFF\tFF\tFF\tFF\tFF\tFF\r\n      1372  1FFFFFFF   00000004    8        00\t00\tFF\tFF\tFF\tFF\tFF\tFF\r\n      1363  0CF102A7   00000004    8        30\t75\tE0\t2E\t80\tFF\tFF\tFD\r\n      1363  0CF101A7   00000004    8        68\t00\t97\tCC\t00\t16\t39\t5E\r\n      1362  1FFFFFFF   00000004    8        00\t00\tFF\tFF\tFF\tFF\tFF\tFF\r\n      1352  1FFFFFFF   00000004    8        00\t00\tFF\tFF\tFF\tFF\tFF\tFF\r\n      1347  1FFFFFFF   00000004    8        00\t20\tFF\tFF\tFF\tFF\tFF\tFF\r\n      1346  18F121F0   00000004    8        09\t18\t00\t00\tFF\tFF\tB0\t01\r\n      1393  18F106A7   00000004    8        00\tF7\tFF\tFF\tFF\tFF\tFF\t8C\r\n      1392  1FFFFFFF   00000004    8        00\t00\tFF\tFF\tFF\tFF\tFF\tFF\r\n      1383  0CF102A7   00000004    8        30\t75\tE0\t2E\t80\tFF\tFF\tFD\r\n      1383  0CF101A7   00000004    8        68\t00\t97\tCC\t00\t16\t39\t5F\r\n      1382  1FFFFFFF   00000004    8        00\t00\tFF\tFF\tFF\tFF\tFF\tFF\r\n      1372  1FFFFFFF   00000004    8        00\t00\tFF\tFF\tFF\tFF\tFF\tFF\r\n      1363  0CF102A7   00000004    8        30\t75\tE0\t2E\t80\tFF\tFF\tFD\r\n      1363  0CF101A7   00000004    8        68\t00\t97\tCC\t00\t16\t39\t5E\r\n      1362  1FFFFFFF   00000004    8        00\t00\tFF\tFF\tFF\tFF\tFF\tFF\r\n      1352  1FFFFFFF   00000004    8        00\t00\tFF\tFF\tFF\tFF\tFF\tFF\r\n      1347  1FFFFFFF   00000004    8        00\t20\tFF\tFF\tFF\tFF\tFF\tFF\r\n      1402  1FFFFFFF   00000004    8        00\t00\tFF\tFF\tFF\tFF\tFF\tFF\r\n      1393  18F106A7   00000004    8        00\tF7\tFF\tFF\tFF\tFF\tFF\t8C\r\n      1392  1FFFFFFF   00000004    8        00\t00\tFF\tFF\tFF\tFF\tFF\tFF\r\n      1383  0CF102A7   00000004    8        30\t75\tE0\t2E\t80\tFF\tFF\tFD\r\n      1383  0CF101A7   00000004    8        68\t00\t97\tCC\t00\t16\t39\t5F\r\n      1382  1FFFFFFF   00000004    8        00\t00\tFF\tFF\tFF\tFF\tFF\tFF\r\n      1372  1FFFFFFF   00000004    8        00\t00\tFF\tFF\tFF\tFF\tFF\tFF\r\n      1363  0CF102A7   00000004    8        30\t75\tE0\t2E\t80\tFF\tFF\tFD\r\n      1363  0CF101A7   00000004    8        68\t00\t97\tCC\t00\t16\t39\t5E\r\n      1362  1FFFFFFF   00000004    8        00\t00\tFF\tFF\tFF\tFF\tFF\tFF\r\n      1352  1FFFFFFF   00000004    8        00\t00\tFF\tFF\tFF\tFF\tFF\tFF\r\n      1403  0CF101A7   00000004    8        68\t00\t97\tCC\t00\t16\t39\t60\r\n      1402  1FFFFFFF   00000004    8        00\t00\tFF\tFF\tFF\tFF\tFF\tFF\r\n      1393  18F106A7   00000004    8        00\tF7\tFF\t
